vi "_Set PIC.vi"(1 "Data":u32) -> (0 "PIC Monitor":u16)   [LabVIEW 2015]
uses:
  <vilib>/rvi/eio/common/nirviEmuTemplateMethod_errors.vi
  <vilib>/rvi/Memory/Memory_Emulation/nirvimemoryEmulation.vi
  <vilib>/rvi/Memory/Memory_Emulation/nirvimemoryFastEmulation.vi
  <vilib>/rvi/DataTransferAndStorage/Container/Common/niFpgaContainerGetUniqueNameForEmu.vi
  <vilib>/rvi/Memory/Memory_Emulation/niFpgaMemoryEmulationCacheClearOnFirstRun.vi
  <vilib>/rvi/Memory/Memory_Emulation/nirvimemoryEmulationManagerCache_MakeExclusive.vi
  <vilib>/rvi/Memory/Memory_Emulation/niFpgaMemoryEmulationValidateCache.vi
  <vilib>/rvi/Memory/Memory_Emulation/nirvimemoryEmulationManagerCache_InsertValue.vi
  <vilib>/Utility/error.llb/Clear Errors.vi
  <vilib>/rvi/Memory/Memory_Emulation/nirvimemoryEmulationManagerCache_ReleaseExclusive.vi
  <vilib>/rvi/Memory/Memory_Emulation/nirvimemoryEmulationManagerCache_GetValue.vi
  <vilib>/rvi/Emulation/niFpgaEmulationIsFPGAContextNoSignature.vi
  <vilib>/rvi/Emulation/niFpgaSctlEmulationGetInTimedLoop.vi
  <vilib>/rvi/Memory/Memory_Emulation/nirvimemoryEmulationManagerCache_SetValue.vi
  <vilib>/rvi/Emulation/niFpgaSctlEmulationResourceMgr.vi
  <vilib>/eio/EIONode/EIONode.xnode
  <vilib>/rvi/DataTransferAndStorage/Container/XNode/niFpgaContainer.xnode
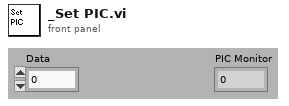
[diagram p1: front panel]
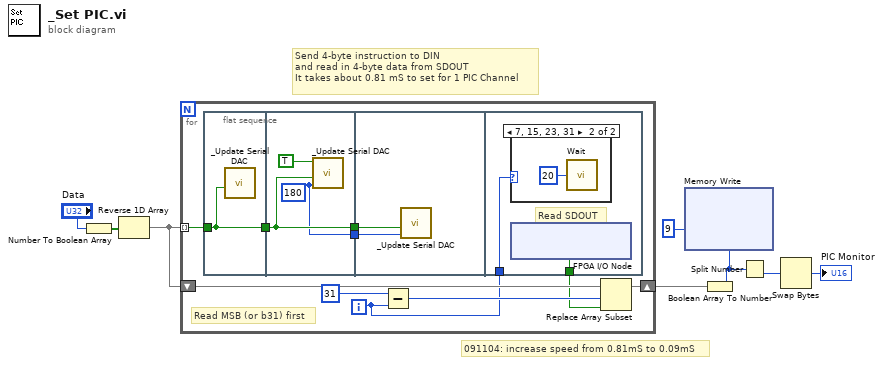
[diagram p0: block diagram]
diagram:
  # "091104: increase speed from 0.81mS to 0.09mS"
  # "Send 4-byte instruction to DIN\nand read in 4-byte data from SDOUT\nIt takes about 0.81 mS to set for 1 PIC Channel"
  n1 = Number To Boolean Array(number="Data") -> (Boolean array=w7:bool[])
  n2 = Reverse 1D Array(array=w7) -> (reversed array=w8:bool[])
  n3 = for {
    shift-right: [w17] -> w4
    shift-left: w8 -> [w18]
    tunnel: w8 -> [w14] mode=indexing
    i -> [w11]
    # "Read MSB (or b31) first"
    n4 = flat-sequence {
      tunnel: w14 -> [w19]
      tunnel: [w19] -> w12
      tunnel: [w21] -> w13
      tunnel: w12 -> [w21]
      tunnel: [w20] -> w9
      tunnel: w13 -> [w24]
      tunnel: w9 -> [w23]
      tunnel: w11 -> [w26]
      tunnel: [w25] -> w10
      frame #0 {
        n5 = call "_Update Serial DAC.vi"("DIN (F)"=w19) -> ()  [unwired: 3 in, 4 out]
      }
      frame #1 {
        w20 = u8 180 ("Wait(12Ticks)")
        n6 = call "_Update Serial DAC.vi"("Wait(12Ticks)"=w20, "DIN (F)"=w21, "Clock (F)"=TRUE) -> ()  [unwired: 1 in, 4 out]
      }
      frame #2 {
        n7 = call "_Update Serial DAC.vi"("Wait(12Ticks)"=w23, "DIN (F)"=w24) -> ()  [unwired: 2 in, 4 out]
      }
      frame #3 {
        # "Read SDOUT"
        n8 = case shown="7, 15, 23, 31" w26 {
          frame 0, Default {
          }
          frame 7, 15, 23, 31 {
            n9 = call "Wait"("Count(uSec)"=u8 20) -> ()  [unwired: 1 out]
          }
        }
        n10 = xnode "FPGA I/O Node"() -> ("Digtal IO/DIO7"=w25:bool)  [unwired: 1 in, 1 out]
      }
    }
    n11 = Subtract(x=31, y=w11) -> (x-y=w15:i32)
    n12 = Replace Array Subset(array=w18, new element=w10, index=w15) -> (w17:bool[])
  }
  n13 = Boolean Array To Number(Boolean array=w4) -> (number=w3:u32)
  n14 = xnode ("Memory Write")("Address"=u8 9, "Data"=w3) -> ()  [unwired: 1 in, 1 out]
  n15 = Split Number(x=w3) -> (lo(x)=w2:u16)  [unwired: 1 out]
  n16 = Swap Bytes(anything=w2) -> (byte swapped=→"PIC Monitor":u16)
